vi "EvaluateDeviceResources.vi"(8 "error in (no error)":errorcluster, 9 "accumulation config":T1, 11 "Qbus":refnum<class "Qbus.lvclass">) -> (0 "error out":errorcluster, 3 "device resources ok":bool)   [LabVIEW 2017, in "DataAccumulator.lvlib"]
uses:
  <vilib>/addons/InsightCM/Devices/Shared/Common/DataAccumulator/DataAccumulator.lvlib
  <vilib>/addons/InsightCM/Devices/Shared/Common/DataAccumulator/controls/config.ctl
  <vilib>/addons/InsightCM/Devices/Shared/Common/DeviceHealth/controls/deviceHealthTag.ctl
  <vilib>/addons/InsightCM/Devices/Shared/Common/DeviceHealth/controls/SystemHealthTagEnum.ctl
  <vilib>/addons/InsightCM/MessageBus/Base/controls/Tag.ctl
  <vilib>/addons/InsightCM/MessageBus/Base/controls/KeyValuePair.ctl
  <vilib>/addons/Qbus/Qbus.lvclass
  <vilib>/addons/SystemInfoProcess/controls/SystemResources.ctl
  <vilib>/addons/SystemInfoProcess/controls/Utilization.ctl
  <vilib>/addons/SystemInfoProcess/controls/CPULoad.ctl
  <vilib>/addons/PointValueMap/subVIs/Point_Read_variant.vi
  <vilib>/addons/SystemInfoProcess/SystemInfoProcess.lvlib
  <vilib>/addons/PointValueMap/PointValueMap.lvlib
  <vilib>/addons/InsightCM/Devices/Shared/Common/DeviceHealth/DeviceHealth.lvlib
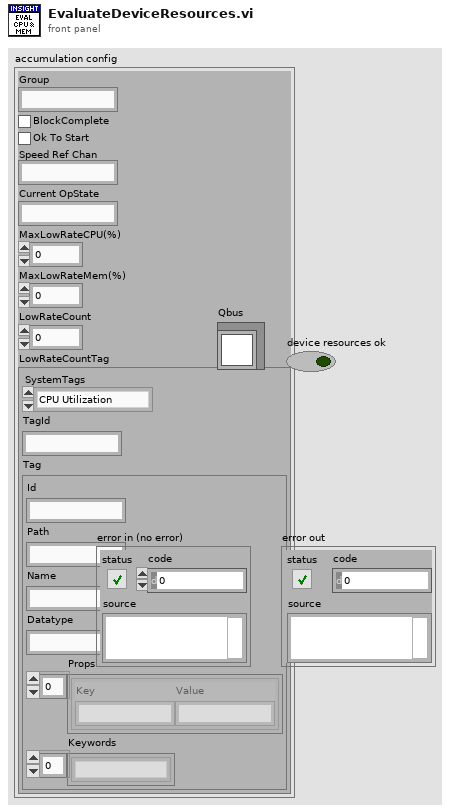
[diagram p1: front panel]
types:
  T1 = typedef "DataAccumulator.lvlib/config.ctl" = cluster{"Group":string, "BlockComplete":bool, "Ok To Start":bool, "Speed Ref Chan":string, "Current OpState":string, "MaxLowRateCPU(%)":dbl, "MaxLowRateMem(%)":dbl, "LowRateCount":i32, "LowRateCountTag":T2}
  T2 = typedef "DeviceHealth.lvlib/deviceHealthTag.ctl" = cluster{"SystemTags":T3, "TagId":string, "Tag":T4}
  T3 = typedef "DeviceHealth.lvlib/SystemHealthTagEnum.ctl" = enum16{"CPU Utilization", "Memory Utilization", "Disk Utilization", "Total Physical Memory", "Primary Disk Free", "Chassis Temperature", "LowRateCount"}
  T4 = typedef "Tag.ctl" = cluster{"Id":string, "Path":string, "Name":string, "Datatype":string, "Props":T5[], "Keywords":string[]}
  T5 = typedef "KeyValuePair.ctl" = cluster{"Key":string, "Value":string}
  T6 = typedef "PointValueMap.lvlib/PointMap.ctl" = refnum<data-value>
  T7 = typedef "SystemInfoProcess.lvlib/SystemResources.ctl" = cluster{"TotalPhysicalMemory":dbl, "FreePhysicalMemory":dbl, "LargestAvailableMemoryBlock":dbl, "TotalVirtualMemory":dbl, "FreeVirtualMemory":dbl, "PrimaryDiskCapacity":dbl, "PrimaryDiskFree":dbl, "Utilization":T8, "CPU Loads":T9[]}
  T8 = typedef "SystemInfoProcess.lvlib/Utilization.ctl" = cluster{"CPU":dbl, "Memory":dbl, "Disk":dbl}
  T9 = typedef "SystemInfoProcess.lvlib/CPULoad.ctl" = cluster{"Total (%)":dbl, "Time Critical (%)":dbl, "Timed Structures (%)":dbl, "High (%)":dbl, "Above Normal (%)":dbl, "Normal (%)":dbl, "Background (%)":dbl, "Idle (%)":dbl, "ISR (%)":dbl}
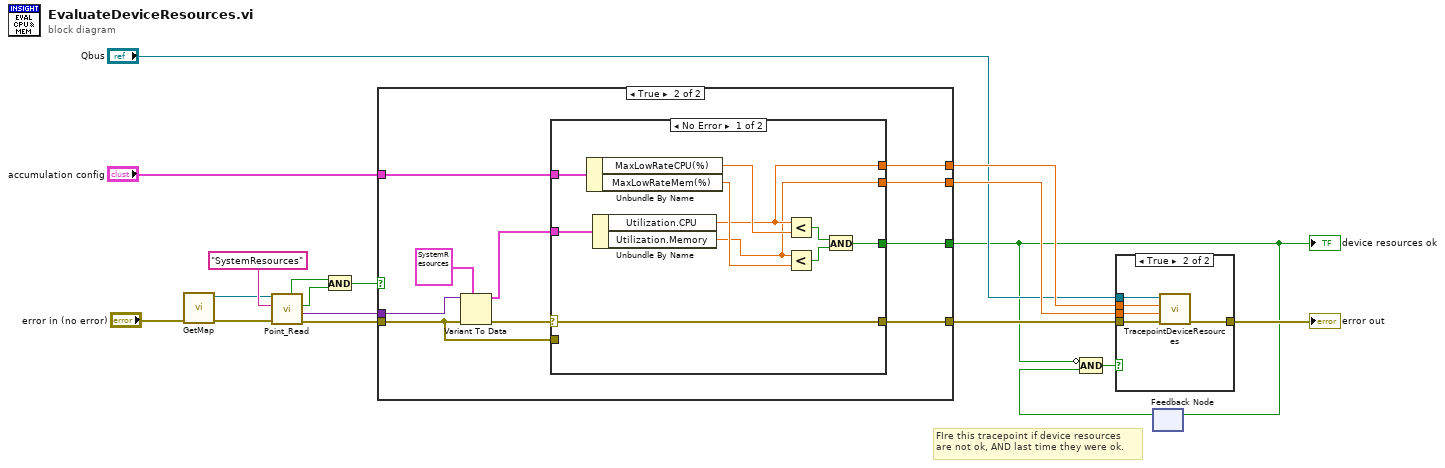
[diagram p0: block diagram]
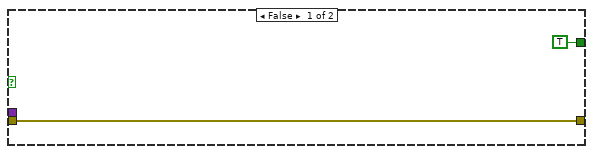
[diagram p3: hidden frame]
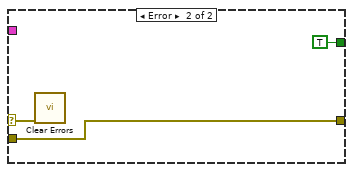
[diagram p4: hidden frame]
diagram:
  # "FIre this tracepoint if device resources\nare not ok, AND last time they were ok."
  n1 = call <vilib>:"GetMap.vi"("error in (no error)"="error in (no error)") -> ("error out"=w14:errorcluster, "SystemInfoMap"=w15:T6)  [unwired: 9 in]
  n2 = call-poly <vilib>:"Point_Read.vi"("Error In"=w14, "Tag"="SystemResources", "Map"=w15) -> ("Error Out"=w13:errorcluster, "Value"=w12:variant, "Found?"=w10:bool, "Valid?"=w9:bool)  [unwired: 3 in, 2 out]
  n3 = And(x=w9, y=w10) -> (x .and. y?=w11:bool)
  n4 = case shown="True" w11 {
    tunnel: w13 -> [w20 w23]
    tunnel: w12 -> [_ w30]
    tunnel: [w20 w28] -> w7
    tunnel: "accumulation config" -> [_ w27]
    tunnel: [TRUE w24] -> w2
    tunnel: [_ w22] -> w6
    tunnel: [_ w21] -> w5
    frame False {
    }
    frame True {
      n5 = Variant To Data(error in=w23, type=T7 {"TotalPhysicalMemory"=0.0, "FreePhysicalMemory"=0.0, "LargestAvailableMemoryBlock"=0.0, "TotalVirtualMemory"=0.0, "FreeVirtualMemory"=0.0, "PrimaryDiskCapacity"=0.0, "PrimaryDiskFree"=0.0, "Utilization"={"CPU"=0.0, "Memory"=0.0, "Disk"=0.0}, "CPU Loads"=[]} ("system resources"), Variant=w30) -> (data=w25:T7, error out=w26:errorcluster)
      n6 = case shown="No Error" w26 {
        selector: w26 -> [w38 w43]
        tunnel: [w38 w41] -> w28
        tunnel: w27 -> [w40 _]
        tunnel: w25 -> [w39 _]
        tunnel: [w35 TRUE] -> w24
        tunnel: w23 -> [_ w41]
        tunnel: [w32 _] -> w22
        tunnel: [w31 _] -> w21
        frame No Error {
          n7 = Unbundle By Name(w40) -> ("MaxLowRateCPU(%)"=w34:dbl, "MaxLowRateMem(%)"=w33:dbl)
          n8 = Unbundle By Name(w39) -> ("Utilization.CPU"=w32:dbl, "Utilization.Memory"=w31:dbl)
          n9 = Less?(x=w32, y=w34) -> (x < y?=w37:bool)
          n10 = Less?(x=w31, y=w33) -> (x < y?=w36:bool)
          n11 = And(x=w37, y=w36) -> (x .and. y?=w35:bool)
        }
        frame Error {
          n12 = call <vilib>:"Clear Errors.vi"("error in (no error)"=w43) -> ()  [unwired: 5 in, 2 out]
        }
      }
    }
  }
  "device resources ok" <- w2
  n13 = feedback #1() -> (w1:bool)  [unwired: 1 in]
  n14 = Compound Arithmetic op=AND(invert w2, w1) -> (w3:bool)
  n15 = case shown="True" w3 {
    tunnel: w7 -> [w44 w49]
    tunnel: [w44 w48] -> w8
    tunnel: "Qbus" -> [_ w47]
    tunnel: w6 -> [_ w46]
    tunnel: w5 -> [_ w45]
    frame False {
    }
    frame True {
      n16 = call <vilib>:"TracepointDeviceResources.vi"("error in (no error)"=w49, "Mem"=w45, "CPU"=w46, "Qbus"=w47) -> ("error out"=w48:errorcluster)  [unwired: 7 in]
    }
  }
  "error out" <- w8
  n17 = feedback-in #1(w2) -> ()
